vi "Run Child.vi"(8 "error in (no error)":errorcluster, 10 "Run Parameters":T1, 11 "Action in":refnum<class "Action.lvclass">) -> (0 "error out":errorcluster, 3 "Action out":refnum<class "Action.lvclass">)   [LabVIEW 2020, in "neg-pkg.lvlib" / "Action.lvclass"]
uses:
  Action.lvclass
  Run Parameters.ctl
  Status/Status.lvclass
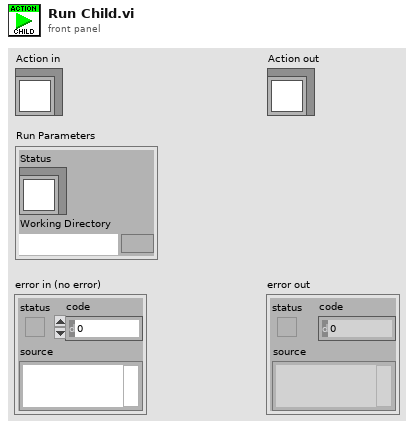
[diagram p1: front panel]
types:
  T1 = typedef "neg-pkg.lvlib/Action.lvclass/Run Parameters.ctl" = cluster{"Status":refnum<class "Status.lvclass">, "Working Directory":path}
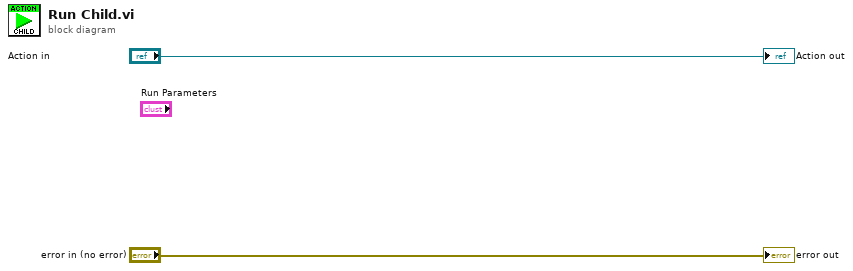
[diagram p0: block diagram]
diagram:
  "error out" <- "error in (no error)"
  "Action out" <- "Action in"
